vi "U32ToSGL.vi"(5 "Number":u32) -> (1 "Single precision float":sgl, 2 "Overflow?":bool, 3 "Exact conversion?":bool)   [LabVIEW 2017, in "GPOverflow.lvlib"]
doc: "Converts <B>Number</B> to SGL keeping track of numeric overflow and exactness of conversion.\n\n<B>Exact conversion?</B> will be True only if a conversion back into the original data type of <B>Number</B> will yield the exact same number, i.e. no precision was lost during the conversion.\n\n<B>Overflow?</B> will be True if positive or negative overflow occurred. The numeric output will saturate in case of overflow.\n\nThis VI is inlined.\n\nSteen Schmidt\nGPower\n7/3 2013"
uses:
  GPOverflow.lvlib
  ToU32/SGLToU32.vi
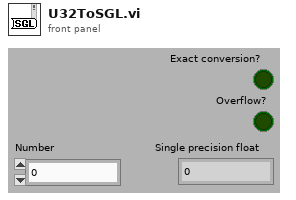
[diagram p1: front panel]
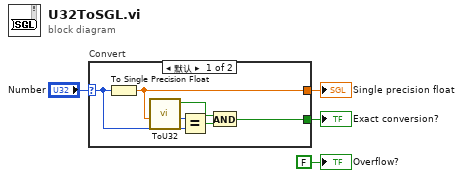
[diagram p0: block diagram]
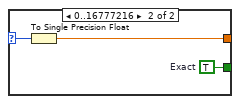
[diagram p2: hidden frame]
diagram:
  n1 = case "Convert" shown="默认" "Number" {
    selector: "Number" -> [w8 w13]
    tunnel: [w10 w12] -> w3
    tunnel: [w5 w11] -> w2
    frame Default {
      n2 = To Single Precision Float(number=w8) -> (single precision float=w10:sgl)
      n3 = call-poly "ToU32.vi"("Number"=w10) -> ("Unsigned 32-bit integer"=w9:u32, "Exact conversion?"=w6:bool)  [unwired: 4 in, 1 out]
      n4 = Equal?(x=w9, y=w8) -> (x = y?=w7:bool)
      n5 = And(x=w6, y=w7) -> (x .and. y?=w5:bool)
    }
    frame 0..16777216 {
      w11 = TRUE  # Exact
      n6 = To Single Precision Float(number=w13) -> (single precision float=w12:sgl)
    }
  }
  "Single precision float" <- w3
  "Exact conversion?" <- w2
  "Overflow?" <- FALSE ("Overflow?")
